vi "Peak Detector (single).vi"(6 "Width Units (points)":enum16{"Points", "Data"}(ring), 8 "error in (no error)":errorcluster, 9 "width":dbl=3.0 min=3.0, 10 "threshold":dbl format="%0.2f", 11 "XY-data":cluster{"X-array":dbl[], "Y-array":dbl[]}) -> (0 "error out":errorcluster, 1 "Amplitudes":dbl[](array[numeric]), 2 "Locations":dbl[](array[numeric]), 3 "XY-data out":cluster{"X-array":dbl[], "Y-array":dbl[]} {"Y-array" format="%.2p"; "X-array" format="%.2p"})   [LabVIEW 2016, in "xy_utilities.lvlib"]
doc: "Find <b>peaks</b> in <b>XY-data</b>'s Y-Array.\n\nWire data to the data input to determine the polymorphic instance to use or manually select the instance."
uses:
  xy_utilities.lvlib
  Private/X Array Range to Index.vi
  <vilib>/Analysis/NI_AAL_SigProc.lvlib
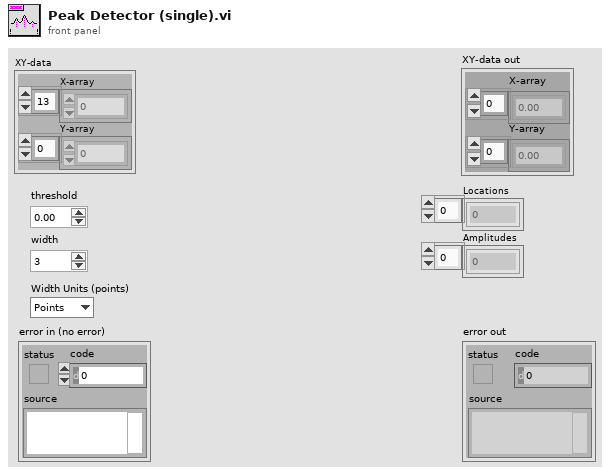
[diagram p1: front panel]
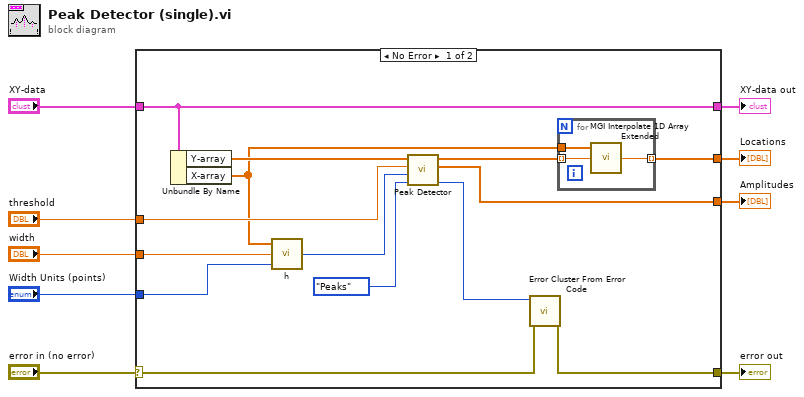
[diagram p0: block diagram]
diagram:
  n1 = case shown="No Error" "error in (no error)" {
    selector: "error in (no error)" -> [w23 w28]
    tunnel: [w22 w28] -> w8
    tunnel: "XY-data" -> [w17 w27]
    tunnel: [w17 w27] -> w6
    tunnel: "threshold" -> [w19 _]
    tunnel: "width" -> [w15 _]
    tunnel: [w10 _] -> w3
    tunnel: [w11 _] -> w2
    tunnel: "Width Units (points)" -> [w16 _]
    frame No Error {
      n2 = Unbundle By Name(w17) -> ("Y-array"=w21:dbl[], "X-array"=w12:dbl[])
      n3 = call "h.vi"("Interval Units (points)"=w16, "Interval (h)"=w15, "X-array"=w12) -> ("h (points)"=w14:i32)
      n4 = call <vilib>:"Peak Detector.vi"("peaks/valleys"=enum32{"Peaks", "Valleys"}."Peaks", "width"=w14, "threshold"=w19, "X"=w21) -> ("error"=w20:i32, "Amplitudes"=w11:dbl[], "Locations"=w13:dbl[])  [unwired: 3 in, 2 out]
      n5 = call <vilib>:"Error Cluster From Error Code.vi"("error in (no error)"=w23, "error code (0)"=w20) -> ("error out"=w22:errorcluster)  [unwired: 7 in]
      n6 = for {
        tunnel: w13 -> [w26] mode=indexing
        tunnel: w12 -> [w25]
        tunnel: [w24] -> w10 mode=indexing
        n7 = call <userlib>:"MGI Interpolate 1D Array Extended.vi"("Fractional X"=w26, "Y Value[]"=w25) -> ("ExtendedY"=w24:dbl)  [unwired: 1 in]
      }
    }
    frame Error {
    }
  }
  "error out" <- w8
  "XY-data out" <- w6
  "Locations" <- w3
  "Amplitudes" <- w2
